vi "bode_ph_offset.vi"() -> ()   [LabVIEW 2014]
doc: "Bode plot\nAcquisisce la risposta di un circuito utilizzando il generatore interno\nGenera il grafico della risposta in funzione della frequenza\nFM & ADL 09/2009, 10/2012, 10/2013 versione per 8.6 \nModifcato con set di DMA e Interrupts FM 10/2013\nversione con offser e ampiezza regolabile"
uses:
  <vilib>/DAQmx/write.llb/DAQmx Write (Analog 1D DBL 1Chan NSamp).vi
  <vilib>/DAQmx/read.llb/DAQmx Read (Analog 1D Wfm NChan NSamp).vi
  <vilib>/DAQmx/create/channels.llb/DAQmx Create Channel (AO-Voltage-Basic).vi
  <vilib>/DAQmx/create/channels.llb/DAQmx Create Channel (AI-Voltage-Basic).vi
  <vilib>/DAQmx/configure/timing.llb/DAQmx Timing (Sample Clock).vi
  <vilib>/DAQmx/miscellaneous.llb/DAQmx Fill In Error Info.vi
  <vilib>/measure/matone.llb/Extract Single Tone Information 1 Chan.vi
  <vilib>/Utility/file.llb/Write To Spreadsheet File (DBL).vi
  <vilib>/measure/NI_MABase.lvlib
  <vilib>/measure/NI_MAPro.lvlib
  <resource>/objmgr/daqmx.rc
panel:
  in  "Guadagno del partitore":dbl=1000.0 format="%_4e"
  in  "FScala Out (33)":dbl(ring)=5.0 items=["10"=10.0, "5"=5.0, "0.5"=0.5, "0.05"=0.05]
  in  "FScala In (68)":dbl(ring)=5.0 items=["10"=10.0, "5"=5.0, "0.5"=0.5, "0.05"=0.05]
  in  "Offset":dbl=-1.02 min=-10.0 max=10.0 step=0.01 format="%.3f"
  in  "Ampiezza":dbl=0.02 format="%.3f"
  out "Foma d'onda generata Vout(t)":waveform(dbl)(graph)
  out "N. misura":i32=20
  in  "SALVA I DATI SU FILE":bool=TRUE caption="ON\nOFF"
  out "Fase":cluster{dbl[], dbl[]}(graph)={[5.0, 6.147467068473125, 7.558270271592312, 9.29284351784663, 11.42548989968722, 14.047564579899898, 17.271388129436826, 21.23505795050611, 26.10836388957094, 32.10006144457005, 39.46681412529165, 48.52418802655607, 59.66016958353027, 73.35178556285486, 90.18553723227052, 110.882524037588, 136.32933299805035, 167.61601701448424, 206.08278894903452, 253.37743168865742, 311.52588344006404, 383.0190218849582, 470.91936472731345, 578.9922573134888, 711.867166947118, 875.2359931869336, 1076.0968890518084, 1323.054037586474, 1626.6862251746509, 2000.0000000000045], [-2.511428467979215, -3.2956057199072006, -7.538567169946305, -10.113388336699302, -10.892831534570234, -13.380062579809533, -10.774958061787402, -13.590987224260658, -21.65618380795769, -25.567045102139673, -29.374990352035297, -30.80584091335669, -40.39456715017832, -46.922681187413104, -49.46128006672848, -55.656601427298085, -62.68913088564615, -64.84436978845952, -67.56276682724092, -74.50767078379593, -76.96614211460007, -77.43816453034884, -79.04548854172731, -83.2980148193289, -80.94888607866157, -84.03334246814163, -78.13471017673413, -78.78110200061434, -92.0554038069169, -84.81527118746277]}
  out "GAIN":cluster{dbl[], dbl[]}(graph)={[5.0, 6.147467068473125, 7.558270271592312, 9.29284351784663, 11.42548989968722, 14.047564579899898, 17.271388129436826, 21.23505795050611, 26.10836388957094, 32.10006144457005, 39.46681412529165, 48.52418802655607, 59.66016958353027, 73.35178556285486, 90.18553723227052, 110.882524037588, 136.32933299805035, 167.61601701448424, 206.08278894903452, 253.37743168865742, 311.52588344006404, 383.0190218849582, 470.91936472731345, 578.9922573134888, 711.867166947118, 875.2359931869336, 1076.0968890518084, 1323.054037586474, 1626.6862251746509, 2000.0000000000045], [0.997344434549249, 0.9962213082665805, 0.9941210435643523, 0.9922479926095603, 0.9878479615556824, 0.9824573247202957, 0.9738931698701306, 0.9613958789343343, 0.9430943055783031, 0.9186590086551807, 0.88260450854282, 0.8371109796491035, 0.7795638387175756, 0.7122020936433959, 0.6364315890190533, 0.5575733199071561, 0.48003430290297966, 0.4070800618335603, 0.3414788103570544, 0.28392605144903055, 0.23469423754251195, 0.19299749424063478, 0.15862845124464225, 0.1302776763618104, 0.10670713632692706, 0.08756567054703944, 0.07027549073207927, 0.057247542713008, 0.0468367874762694, 0.03824708830461569]}
  out "Foma d'onda generata Vin(t)":waveform(dbl)(graph)
  out "f_attuale":dbl=2000.0000000000045
  in  "Ncamp/periodo":dbl=25.0
  in  "Nperiodi":dbl=5.0
  in  "Numero misure":i16=30
  in  "Freqmax":dbl=2000.0 max=100000.0
  in  "Freqmin":dbl=5.0
  # "1) Scegliere l'intervallo di frequenza (max 8 kHz) e il numero di misure.\n2) Scegliere quanti periodi della sinusoide si prendono e quanti campioni si generano per ogni periodo; per le frequenze alte ridurre il NCamp/periodo: il prodotto Fmax * Ncamp non deve superare  ~ 60000.\n3) Premere la freccia bianca di avvio."
  # "Fase"
  # "I Collegamenti"
  # "Collegare il CB 22 (Analog Output 0) all'ingresso. \nI due canali di misura (riferiti a terra) sono il CB68 (Vin) e CB33 (Vout).\nLa terra del circuito DEVE essere in comune alla terra della scheda (CB29)."
  # "NO\nSI"
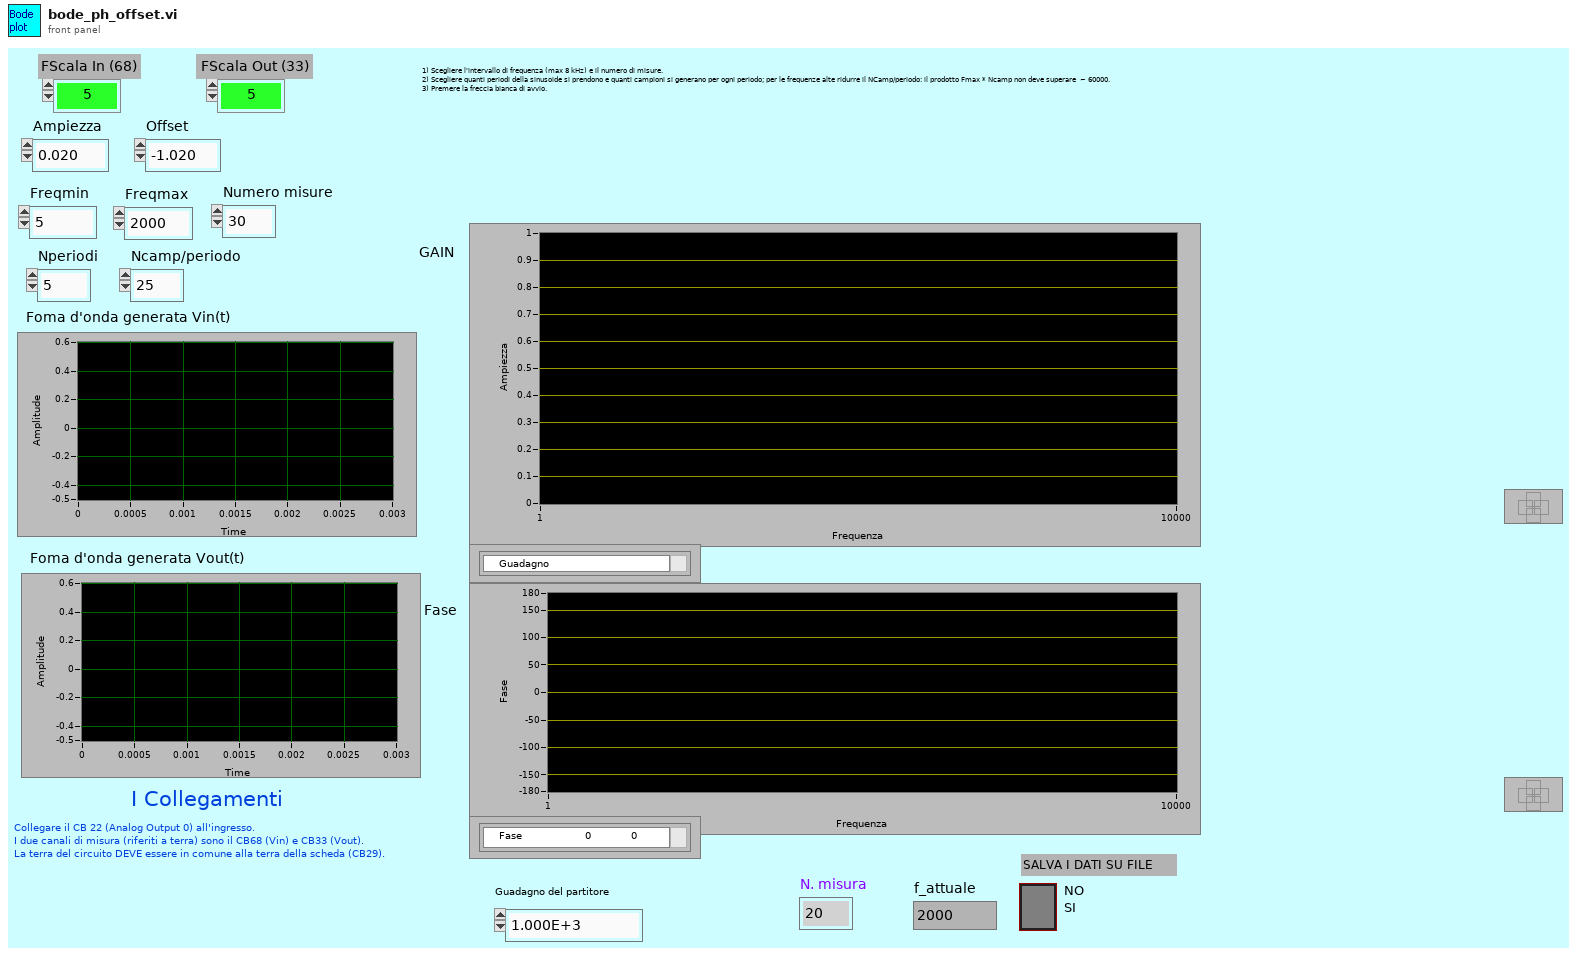
[diagram p1: front panel]
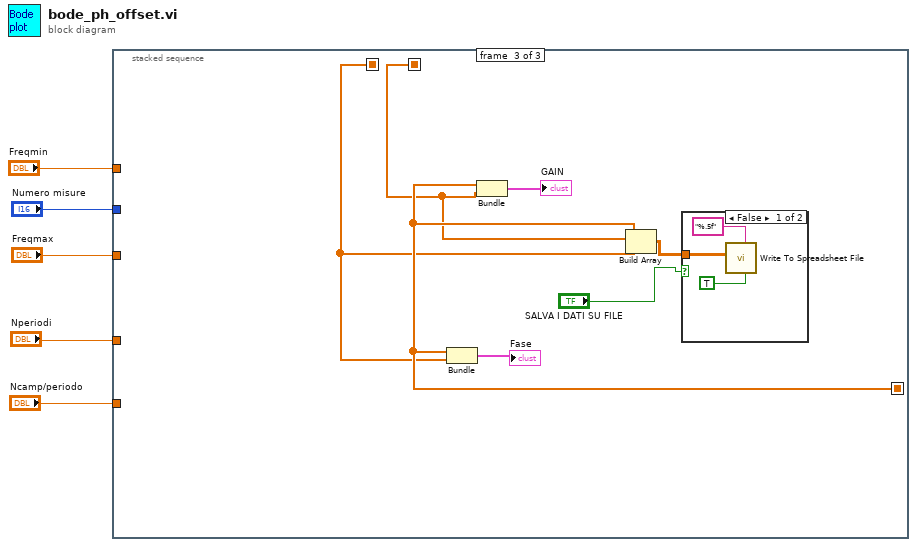
[diagram p0: block diagram]
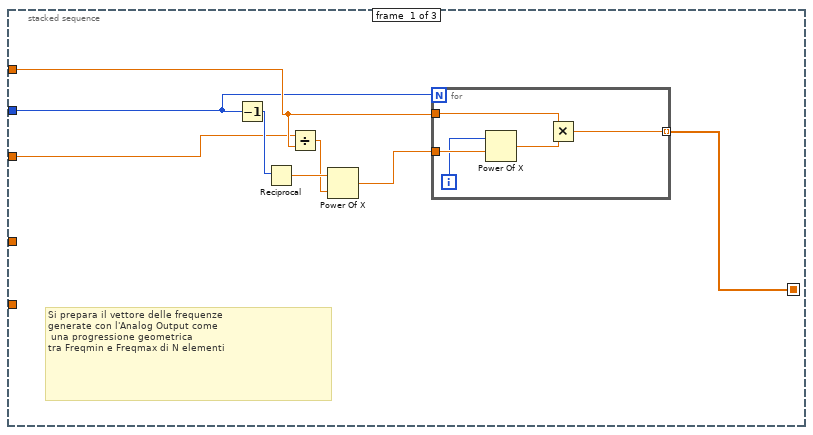
[diagram p2: hidden frame]
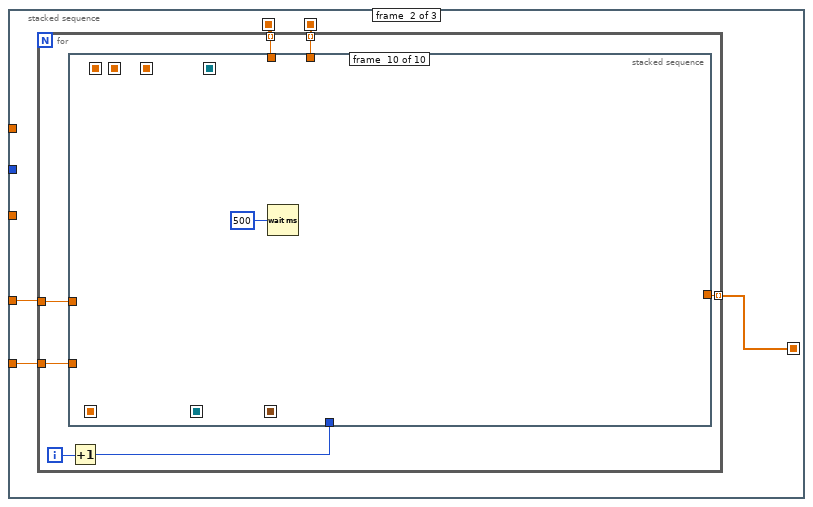
[diagram p3: hidden frame]
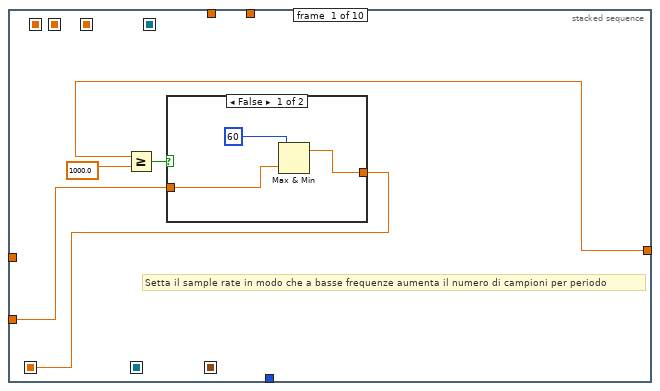
[diagram p4: hidden frame]
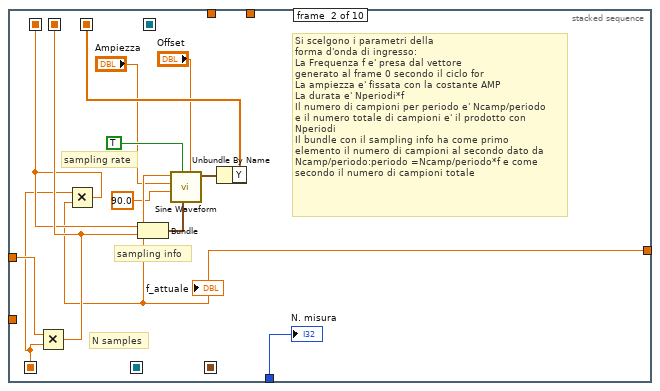
[diagram p6: hidden frame]
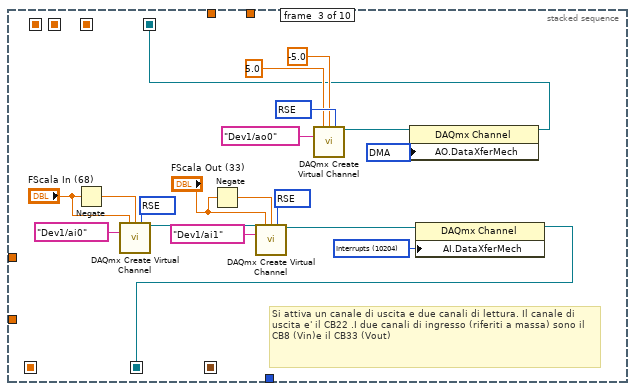
[diagram p7: hidden frame]
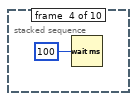
[diagram p8: hidden frame]
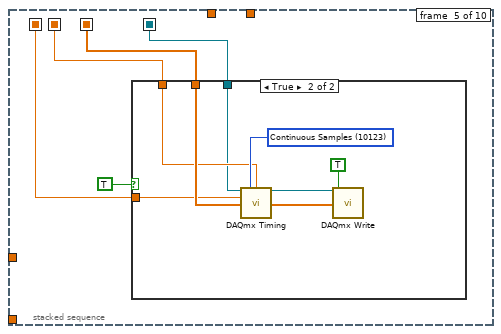
[diagram p9: hidden frame]
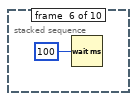
[diagram p11: hidden frame]
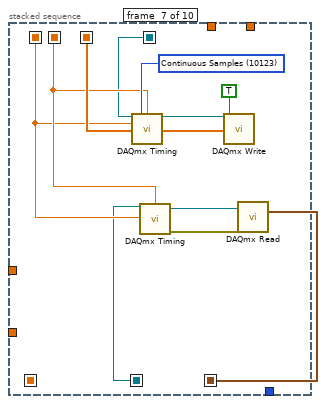
[diagram p12: hidden frame]
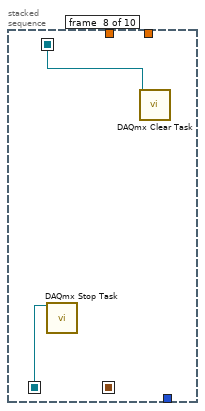
[diagram p13: hidden frame]
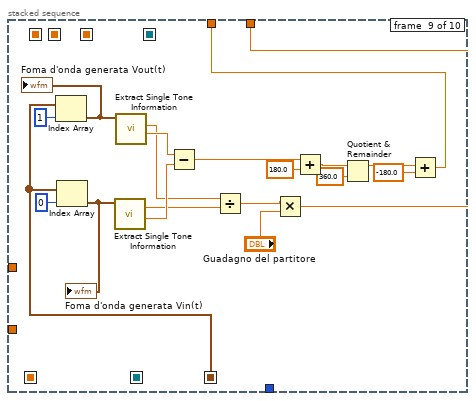
[diagram p14: hidden frame]
diagram:
  n1 = stacked-sequence {
    seq-local: [w6 _ _] -> [_ w22 w123]
    seq-local: [_ w19 _] -> [_ _ w122]
    seq-local: [_ w20 _] -> [_ _ w121]
    tunnel: "Freqmin" -> [w9 _ _]
    tunnel: "Numero misure" -> [w8 _ _]
    tunnel: "Freqmax" -> [w7 _ _]
    tunnel: "Ncamp/periodo" -> [_ w23 _]
    tunnel: "Nperiodi" -> [_ w21 _]
    frame #0 {
      # "Si prepara il vettore delle frequenze\ngenerate con l'Analog Output come\n una progressione geometrica\ntra Freqmin e Freqmax di N elementi"
      n2 = Decrement(x=w8) -> (x-1=w13:i16)
      n3 = Reciprocal(x=w13) -> (1/x=w12:dbl)
      n4 = Divide(x=w7, y=w9) -> (x/y=w11:dbl)
      n5 = Power Of X(1:w11, 2:w12) -> (0:w10:dbl)
      n6 = for {
        N: w8 -> [_]
        tunnel: w10 -> [w18]
        tunnel: w9 -> [w16]
        tunnel: [w14] -> w6 mode=indexing
        i -> [w17]
        n7 = Power Of X(1:w18, 2:w17) -> (0:w15:dbl)
        n8 = Multiply(x=w16, y=w15) -> (x*y=w14:dbl)
      }
    }
    frame #1 {
      n9 = for {
        tunnel: w23 -> [w30]
        tunnel: w22 -> [w27] mode=indexing
        tunnel: w21 -> [w29]
        tunnel: [w28] -> w20 mode=indexing
        tunnel: [w24] -> w19 mode=indexing
        i -> [w26]
        n10 = Increment(x=w26) -> (x+1=w25:i32)
        n11 = stacked-sequence {
          seq-local: [_ w51 _ _ _ _ _ _ _ _] -> [_ _ _ _ w77 _ w91 _ _ _]
          seq-local: [_ w48 _ _ _ _ _ _ _ _] -> [_ _ _ _ w76 _ w89 _ _ _]
          seq-local: [_ w47 _ _ _ _ _ _ _ _] -> [_ _ _ _ w75 _ w88 _ _ _]
          seq-local: [_ _ _ _ _ _ w92 _ _ _] -> [_ _ _ _ _ _ _ _ w117 _]
          seq-local: [w31 _ _ _ _ _ _ _ _ _] -> [_ w43 _ _ _ _ _ _ _ _]
          seq-local: [_ _ w63 _ _ _ _ _ _ _] -> [_ _ _ _ w74 _ w87 w97 _ _]
          seq-local: [_ _ w61 _ _ _ _ _ _ _] -> [_ _ _ _ _ _ w86 w98 _ _]
          tunnel: w30 -> [w32 _ _ _ _ _ _ _ _ _]
          tunnel: w27 -> [w35 w46 _ _ _ _ _ _ _ _]
          tunnel: w29 -> [_ w49 _ _ _ _ _ _ _ _]
          tunnel: [_ _ _ _ _ _ _ _ w104 _] -> w28
          tunnel: w25 -> [_ w42 _ _ _ _ _ _ _ _]
          tunnel: [_ _ _ _ _ _ _ _ w99 _] -> w24
          frame #0 {
            # "Setta il sample rate in modo che a basse frequenze aumenta il numero di campioni per periodo"
            n12 = Greater Or Equal?(x=w35, y=1000.0) -> (x >= y?=w33:bool)
            n13 = case shown="False" w33 {
              tunnel: [w36 w39] -> w31
              tunnel: w32 -> [w37 w39]
              frame False {
                n14 = Max & Min(x=60, y=w37) -> (max(x,y)=w36:dbl)  [unwired: 1 out]
              }
              frame True {
              }
            }
          }
          frame #1 {
            # "Si scelgono i parametri della\nforma d'onda di ingresso:\nLa Frequenza f e' presa dal vettore \ngenerato al frame 0 secondo il ciclo for\nLa ampiezza e' fissata con la costante AMP\nLa durata e' Nperiodi*f\nIl numero di campioni per periodo e' Ncamp/periodo\ne il numero totale di campioni e' il prodotto con \nNperiodi\nIl bundle con il sampling info ha come primo\nelemento il numero di campioni al secondo dato da \nNcamp/periodo:periodo =Ncamp/periodo*f e come\nsecondo il numero di campioni totale"
            # "sampling rate"
            # "N samples"
            # "sampling info"
            n15 = Multiply(x=w49, y=w43) -> (x*y=w48:dbl)
            n16 = Multiply(x=w43, y=w46) -> (x*y=w47:dbl)
            n17 = Bundle(w47, w48) -> (w50:cluster{dbl, dbl})  [unwired: 1 out]
            n18 = call <vilib>:"Sine Waveform.vi"("offset"="Offset", "sampling info"=w50, "reset signal"=TRUE, "phase"=90.0, "amplitude"="Ampiezza", "frequency"=w46) -> ("signal out"=w52:waveform(dbl))  [unwired: 1 in, 4 out]
            n19 = Unbundle By Name(w52) -> ("Y"=w51:dbl[])
            "f_attuale" <- w46
            "N. misura" <- w42
          }
          frame #2 {
            w57 = 10083 items=["default"=-1, "RSE"=10083, "NRSE"=10078, "Differential"=10106, "Pseudodifferential"=12529] ("input terminal configuration")
            w62 = 10204 items=["DMA"=10054, "Interrupts"=10204, "Programmed I/O"=10264, "USB Bulk"=12590] ("AO.DataXferMech")
            w65 = 10054 items=["DMA"=10054, "Interrupts"=10204, "Programmed I/O"=10264, "USB Bulk"=12590] ("AO.DataXferMech")
            w66 = 10083 items=["default"=-1, "RSE"=10083, "NRSE"=10078, "Differential"=10106, "Pseudodifferential"=12529] ("input terminal configuration")
            w70 = 10083 items=["Default"=-1, "RSE"=10083, "Differential"=10106, "Pseudodifferential"=12529] ("output terminal configuration")
            # "Si attiva un canale di uscita e due canali di lettura. Il canale di uscita e' il CB22 .I due canali di ingresso (riferiti a massa) sono il CB8 (Vin)e il CB33 (Vout)"
            n20 = Negate(x="FScala In (68)") -> (-x=w60:dbl)
            n21 = call-poly <vilib>:"DAQmx Create Virtual Channel.vi"("maximum value"="FScala In (68)", "minimum value"=w60, "input terminal configuration"=w66, "physical channels"=tag "Dev1/ai0") -> ("task out"=w54:refnum<k21>)  [unwired: 5 in, 6 out]
            n22 = Negate(x="FScala Out (33)") -> (-x=w56:dbl)
            n23 = call-poly <vilib>:"DAQmx Create Virtual Channel.vi"("task in"=w54, "maximum value"="FScala Out (33)", "minimum value"=w56, "input terminal configuration"=w57, "physical channels"=tag "Dev1/ai1") -> ("task out"=w53:refnum<k21>)  [unwired: 4 in, 6 out]
            n24 = call-poly <vilib>:"DAQmx Create Virtual Channel.vi"("maximum value"=5.0, "minimum value"=-5.0, "output terminal configuration"=w70, "physical channels"=tag "Dev1/ao0") -> ("task out"=w64:refnum<k21>)  [unwired: 5 in, 6 out]
            n25 = property class="DAQmx Channel"(reference=w64, "AO.DataXferMech"=w65) -> (reference out=w63:refnum<k21>)  [unwired: 1 in, 1 out]
            n26 = property class="DAQmx Channel"(reference=w53, "AI.DataXferMech"=w62) -> (reference out=w61:refnum<k21>)  [unwired: 1 in, 1 out]
          }
          frame #3 {
            n27 = Wait (ms)(milliseconds to wait=u32 100 ("millisecond multiple")) -> ()  [unwired: 1 out]
          }
          frame #4 {
            n28 = case shown="True" TRUE {
              tunnel: w77 -> [_ w82]
              tunnel: w76 -> [_ w80]
              tunnel: w75 -> [_ w79]
              tunnel: w74 -> [_ w78]
              frame False {
              }
              frame True {
                w81 = 10123 items=["Finite Samples"=10178, "Continuous Samples"=10123, "Hardware Timed Single Point"=12522] ("sample mode")
                n29 = call-poly <vilib>:"DAQmx Timing.vi"("task/channels in"=w78, "sample mode"=w81, "samples per channel"=w80, "rate"=w79) -> ("task out"=w83:refnum<k21>)  [unwired: 3 in, 8 out]
                n30 = call-poly <vilib>:"DAQmx Write.vi"("task/channels in"=w83, "auto start"=TRUE, "data"=w82) -> ()  [unwired: 1 in, 12 out]
              }
            }
          }
          frame #5 {
            n31 = Wait (ms)(milliseconds to wait=u32 100 ("millisecond multiple")) -> ()  [unwired: 1 out]
          }
          frame #6 {
            w90 = 10123 items=["Finite Samples"=10178, "Continuous Samples"=10123, "Hardware Timed Single Point"=12522] ("sample mode")
            n32 = call-poly <vilib>:"DAQmx Timing.vi"("task/channels in"=w87, "sample mode"=w90, "samples per channel"=w89, "rate"=w88) -> ("task out"=w93:refnum<k21>)  [unwired: 3 in, 8 out]
            n33 = call-poly <vilib>:"DAQmx Timing.vi"("task/channels in"=w86, "samples per channel"=w89, "rate"=w88) -> ("task out"=w96:refnum<k21>, "error out"=w95:errorcluster)  [unwired: 4 in, 7 out]
            n34 = call-poly <vilib>:"DAQmx Write.vi"("task/channels in"=w93, "auto start"=TRUE, "data"=w91) -> ()  [unwired: 1 in, 12 out]
            n35 = call-poly <vilib>:"DAQmx Read.vi"("task/channels in"=w96, "error in"=w95) -> ("data"=w92:waveform(dbl)[])  [unwired: 1 in, 12 out]
          }
          frame #7 {
            n36 = call <vilib>:"DAQmx Stop Task.vi"("task/channels in"=w98) -> ()  [unwired: 1 in, 14 out]
            n37 = call <vilib>:"DAQmx Clear Task.vi"("task in"=w97) -> ()  [unwired: 1 in, 14 out]
          }
          frame #8 {
            n38 = Index Array(array=w117, index=1) -> (element=w102:waveform(dbl))
            "Foma d'onda generata Vout(t)" <- w102
            n39 = Index Array(array=w117, index=0) -> (element=w103:waveform(dbl))
            "Foma d'onda generata Vin(t)" <- w103
            n40 = call-poly <vilib>:"Extract Single Tone Information.vi"("time signal in"=w103) -> ("detected phase (deg)"=w114:dbl, "detected amplitude"=w111:dbl)  [unwired: 3 in, 6 out]
            n41 = call-poly <vilib>:"Extract Single Tone Information.vi"("time signal in"=w102) -> ("detected phase (deg)"=w115:dbl, "detected amplitude"=w112:dbl)  [unwired: 3 in, 6 out]
            n42 = Subtract(x=w115, y=w114) -> (x-y=w105:dbl)
            n43 = Divide(x=w112, y=w111) -> (x/y=w101:dbl)
            n44 = Multiply(x=w101, y="Guadagno del partitore") -> (x*y=w99:dbl)
            n45 = Add(x=w105, y=180.0) -> (x+y=w107:dbl)
            n46 = Quotient & Remainder(x=w107, y=360.0) -> (x-y*floor(x/y)=w109:dbl)  [unwired: 1 out]
            n47 = Add(x=w109, y=-180.0) -> (x+y=w104:dbl)
          }
          frame #9 {
            n48 = Wait (ms)(milliseconds to wait=u32 500 ("millisecond multiple")) -> ()  [unwired: 1 out]
          }
        }
      }
    }
    frame #2 {
      n49 = Bundle(w123, w121) -> (→"Fase":cluster{dbl[], dbl[]})  [unwired: 1 out]
      n50 = Bundle(w123, w122) -> (→"GAIN":cluster{dbl[], dbl[]})  [unwired: 1 out]
      n51 = Build Array(w123, w122, w121) -> (w120:dbl[][])
      n52 = case shown="False" "SALVA I DATI SU FILE" {
        tunnel: w120 -> [w128 _]
        frame False {
          n53 = call-poly <vilib>:"Write To Spreadsheet File.vi"("transpose? (no:F)"=TRUE, "format (%.3f)"="%.5f", "2D data"=w128) -> ()  [unwired: 3 in, 3 out]
        }
        frame True {
        }
      }
    }
  }
